vi "Refresh Hierarchy View.vi"(8 "Error in":errorcluster caption="Error in (no error)", 11 "Tree":refnum<vi>) -> (0 "Error out":errorcluster)   [LabVIEW 2018]
uses:
  TypeDef/Refresh Hierarchy View - States.ctl
  TypeDef/BOM Table Raw Items.ctl
  TypeDef/FIlter.ctl
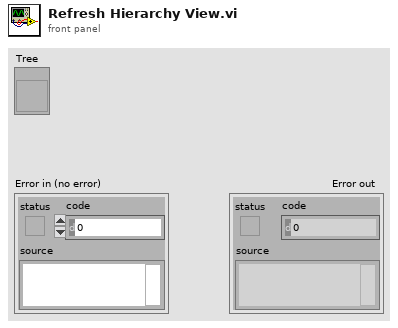
[diagram p1: front panel]
types:
  T1 = typedef "BOM Table Raw Items.ctl" = cluster{"id":i32, "Full PN":string, "External Part Number":string, "Item description":string, "Part Number":string, "Revision":string, "Containing":cluster{"id":i32, "value":string}[], "Contained by":cluster{"id":i32, "value":string}[], "Part of a set":cluster{"id":i32}[]}
  T2 = typedef "Refresh Hierarchy View - States.ctl" = enum16{"Defer Panel Updates", "Cleanup Tree", "Set Up Columns", "Ping API", "GET BOM Rows", "Populate Table", "Adjust Column Width", "Release Panel Updates", "Report Error", "Exit"}
  T3 = typedef "FIlter.ctl" = cluster{"Field Name":string, "Filter Type":string, "Filter Value":string}
  T4 = cluster{"ID":i32, "Item":cluster{"id":i32}[], "Contains":cluster{"id":i32}[], "Amount of Times":string, "Length (mm)":string}
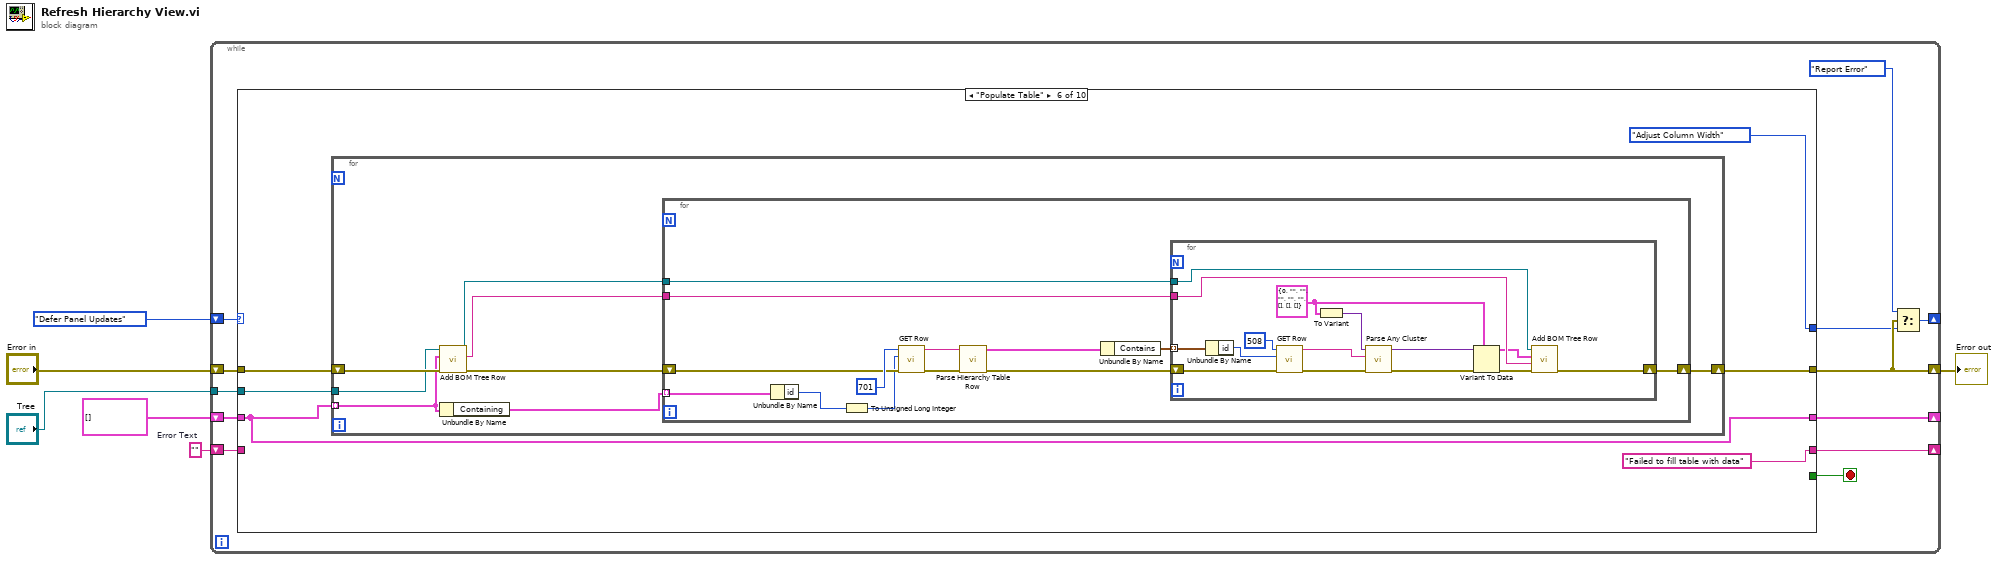
[diagram p0: block diagram]
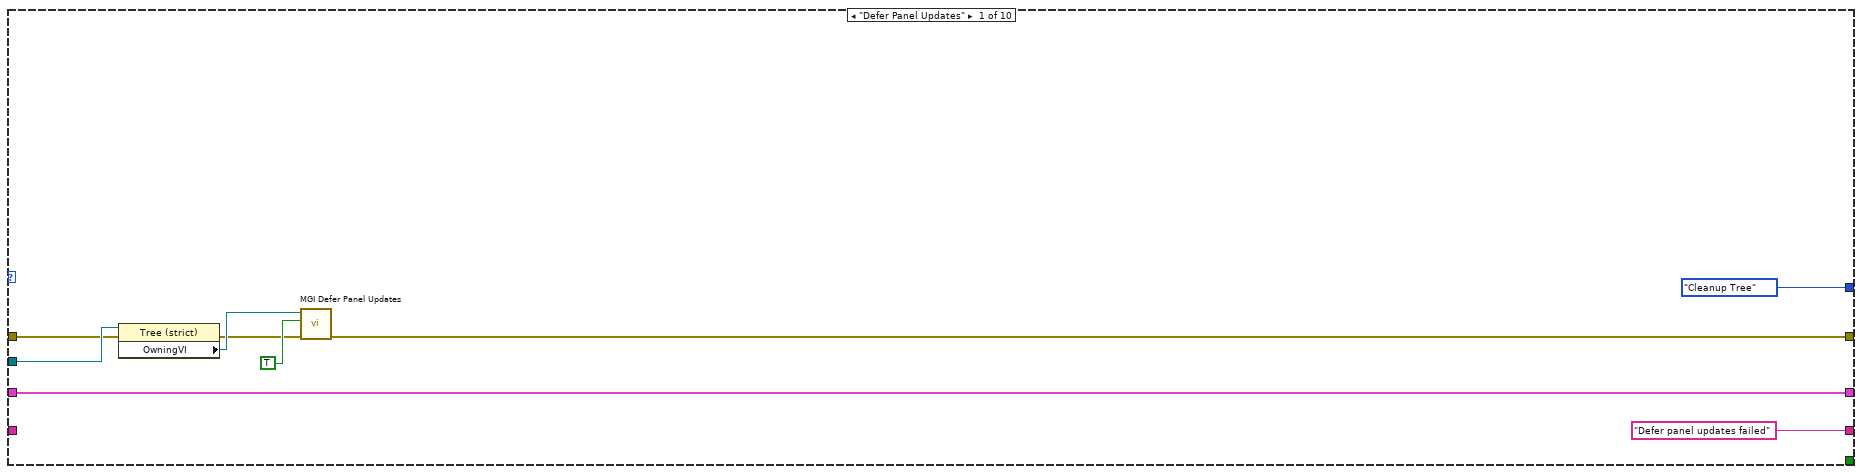
[diagram p2: hidden frame]
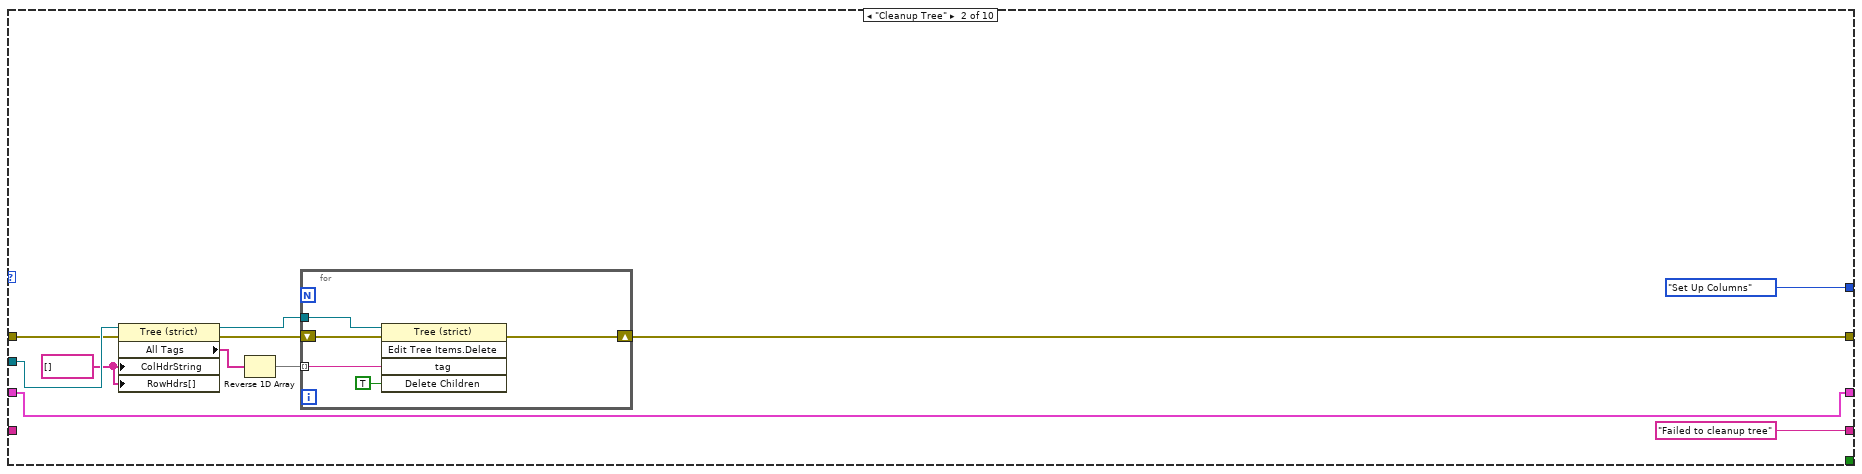
[diagram p3: hidden frame]
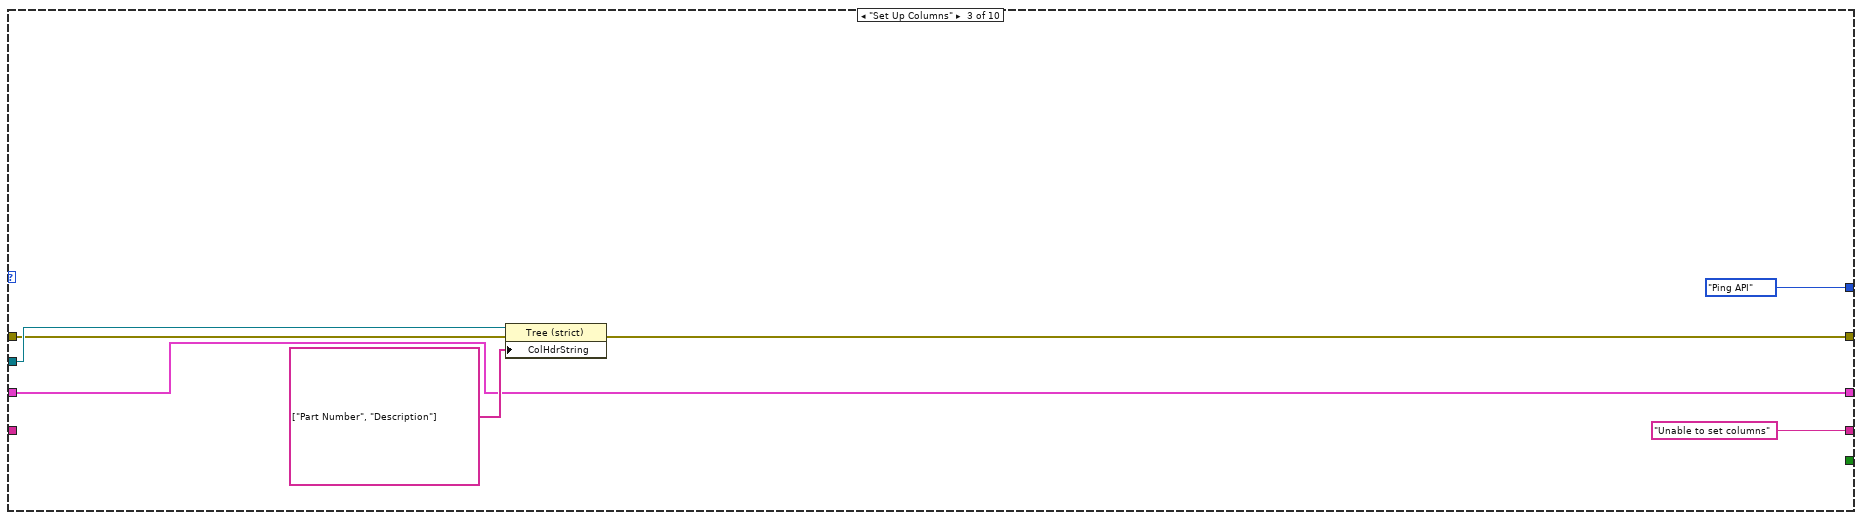
[diagram p4: hidden frame]
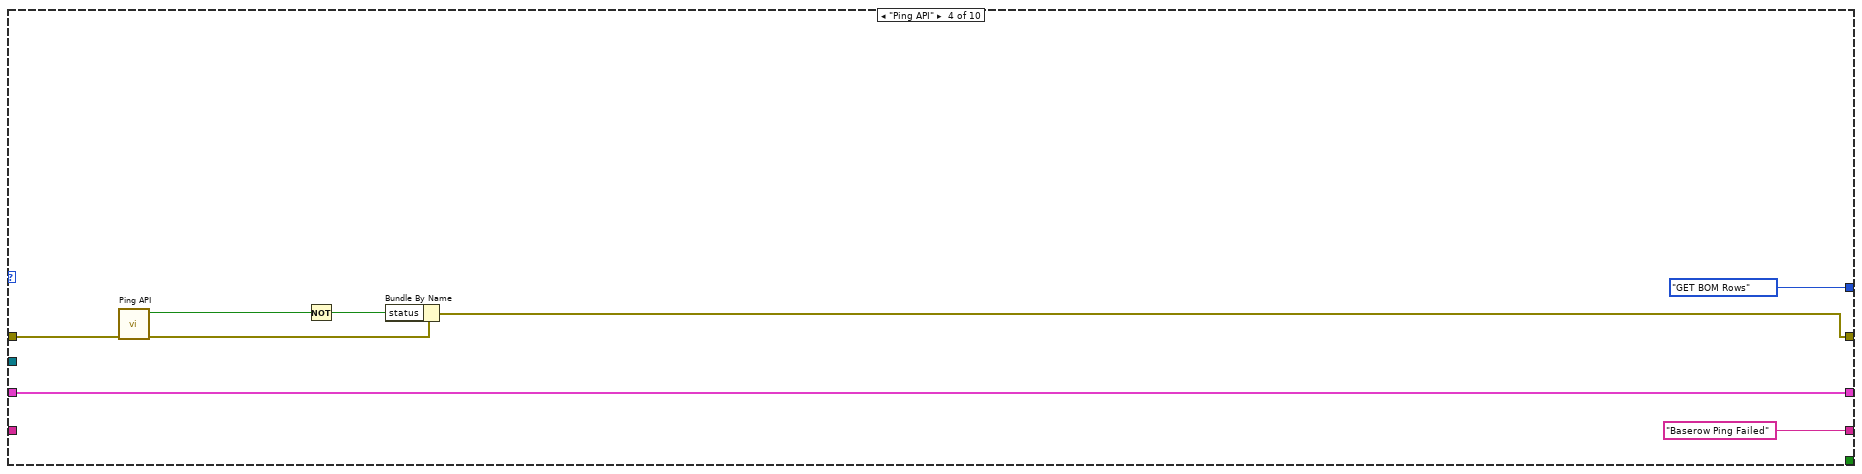
[diagram p5: hidden frame]
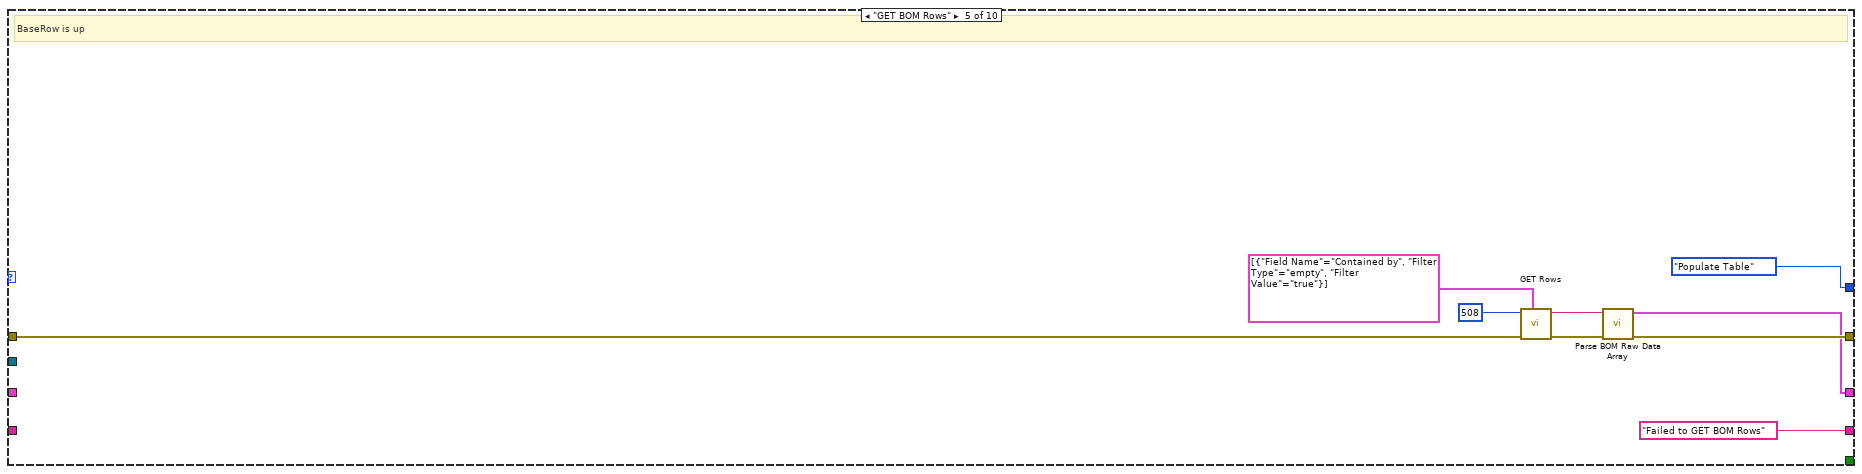
[diagram p6: hidden frame]
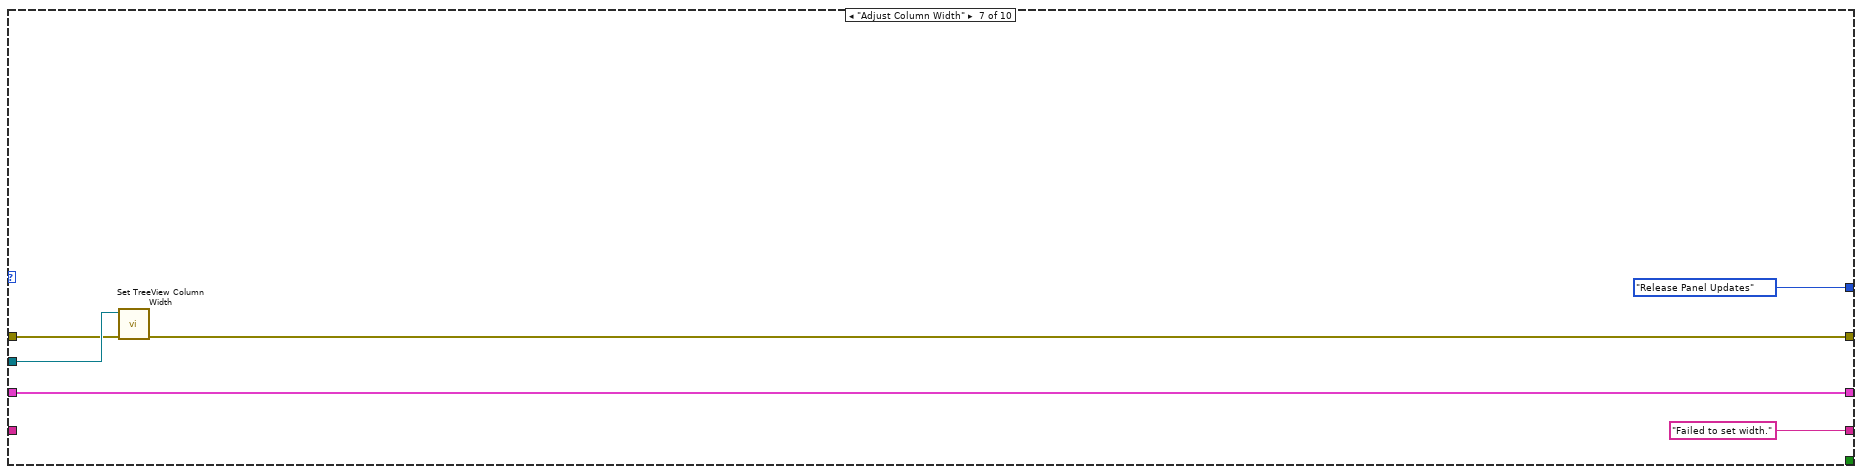
[diagram p7: hidden frame]
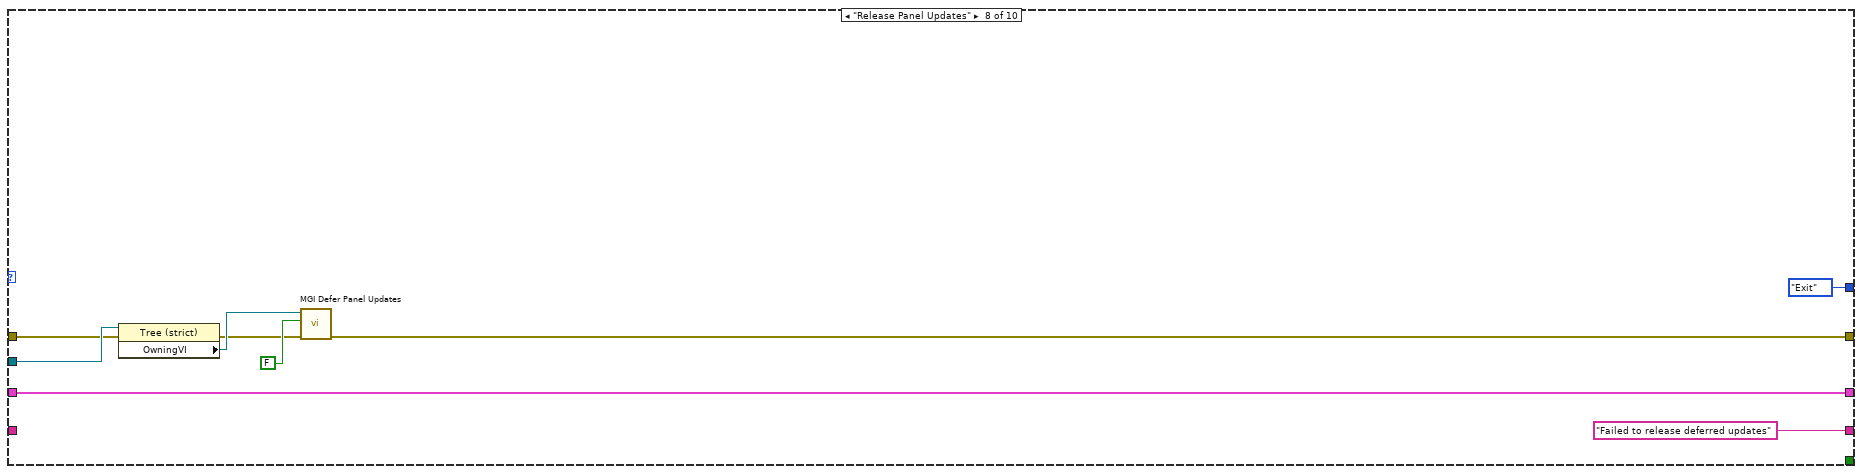
[diagram p8: hidden frame]
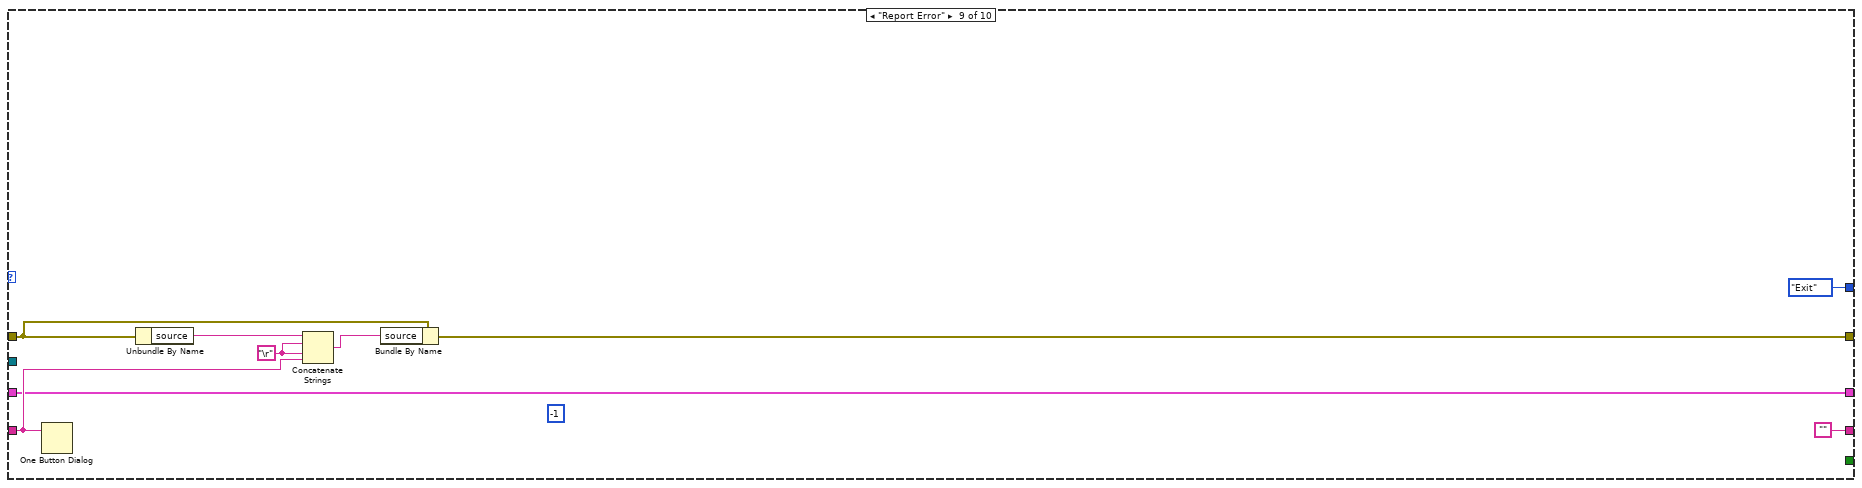
[diagram p9: hidden frame]
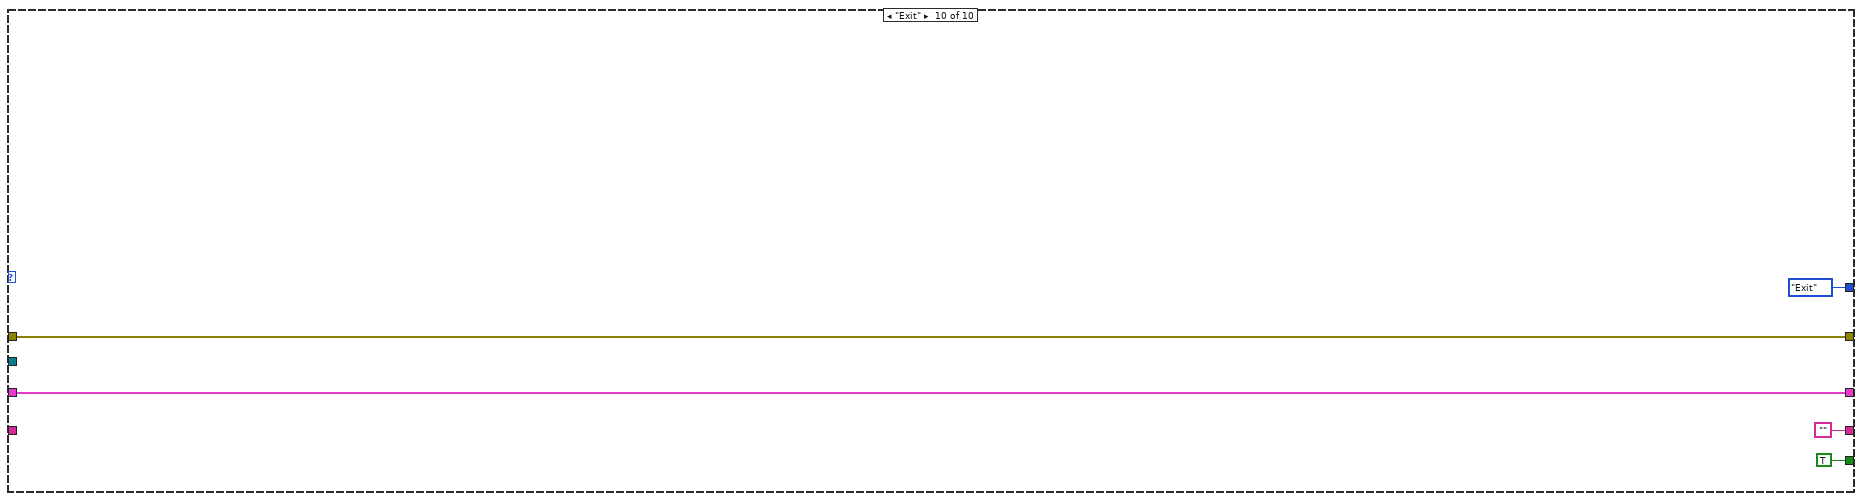
[diagram p10: hidden frame]
diagram:
  w3 = ""  # Error Text
  n1 = while {
    shift-right: [w13] -> w6
    shift-left: "Error in" -> [w17]
    tunnel: "Tree" -> [w14]
    shift-right: [w11] -> _
    shift-left: Refresh_Hierarchy_View_-_States."Defer Panel Updates" -> [w18]
    shift-right: [w9] -> _
    shift-left: w3 -> [w15]
    shift-right: [w8] -> _
    shift-left: T1[] [] ("BOM Items Raw Data") -> [w7]
    stop <- w16 stop-if-true
    n2 = case shown="\"Populate Table\"" w18 {
      tunnel: [w24 w32 w49 w56 w62 w71 w111 w121 w132 w137] -> w13
      tunnel: w17 -> [w22 w37 w48 w58 w65 w70 w110 w119 w131 w137]
      tunnel: [_ _ _ _ _ _ _ _ _ TRUE] -> w16
      tunnel: w15 -> [_ _ _ _ _ _ _ _ w128 _]
      tunnel: w14 -> [w27 w38 w50 _ _ w72 w112 w124 _ _]
      tunnel: [Refresh_Hierarchy_View_-_States."Cleanup Tree" Refresh_Hierarchy_View_-_States."Set Up Columns" Refresh_Hierarchy_View_-_States."Ping API" Refresh_Hierarchy_View_-_States."GET BOM Rows" Refresh_Hierarchy_View_-_States."Populate Table" Refresh_Hierarchy_View_-_States."Adjust Column Width" Refresh_Hierarchy_View_-_States."Release Panel Updates" Refresh_Hierarchy_View_-_States."Exit" Refresh_Hierarchy_View_-_States."Exit" Refresh_Hierarchy_View_-_States."Exit"] -> w12
      tunnel: ["Defer panel updates failed" "Failed to cleanup tree" "Unable to set columns" "Baserow Ping Failed" "Failed to GET BOM Rows" "Failed to fill table with data" "Failed to set width." "Failed to release deferred updates" "" ""] -> w9
      tunnel: [w19 w28 w44 w51 w59 w68 w115 w117 w125 w134] -> w8
      tunnel: w7 -> [w19 w28 w44 w51 _ w68 w115 w117 w125 w134]
      frame "Defer Panel Updates" {
        n3 = property class="Tree (strict)"(reference=w27, error in=w22) -> (error out=w23:errorcluster, "OwningVI"=w26:refnum<vi>)  [unwired: 1 out]
        n4 = call <userlib>:"MGI Defer Panel Updates.vi"("Error In"=w23, "Defer Updates?"=TRUE, "VI Reference (Caller)"=w26) -> ("Error Out"=w24:errorcluster)  [unwired: 8 in]
      }
      frame "Cleanup Tree" {
        w31 = string[] [] ("Column Header Strings[]")
        n5 = property class="Tree (strict)"(reference=w38, error in=w37, "ColHdrString"=w31, "RowHdrs[]"=w31) -> (reference out=w35:refnum<vi>, error out=w33:errorcluster, "All Tags"=w36:string[])
        n6 = Reverse 1D Array(array=w36) -> (reversed array=w34:string[])
        n7 = for {
          tunnel: w35 -> [w43]
          tunnel: w34 -> [w42] mode=indexing
          shift-right: [w39] -> w32
          shift-left: w33 -> [w40]
          n8 = invoke class="Tree (strict)" method="Edit Tree Items.Delete"(reference=w43, error in=w40, "tag"=w42, "Delete Children"=TRUE ("Delete Children?")) -> (error out=w39:errorcluster)  [unwired: 1 in, 4 out]
        }
      }
      frame "Set Up Columns" {
        n9 = property class="Tree (strict)"(reference=w50, error in=w48, "ColHdrString"=string[] ["Part Number", "Description"] ("Column Header Strings[]")) -> (error out=w49:errorcluster)  [unwired: 1 out]
      }
      frame "Ping API" {
        n10 = call "Ping API.vi"("Error in"=w58) -> ("Error out"=w57:errorcluster, "Connection OK"=w55:bool)  [unwired: 9 in]
        n11 = Not(x=w55) -> (.not. x?=w52:bool)
        n12 = Bundle By Name(cluster=w57, "status"=w52) -> (w56:errorcluster)
      }
      frame "GET BOM Rows" {
        # "BaseRow is up"
        n13 = call "GET Rows.vi"("Filters"=T3[] [{"Field Name"="Contained by", "Filter Type"="empty", "Filter Value"="true"}], "Error in"=w65, "Table ID"=u32 508) -> ("Error out"=w63:errorcluster, "Rows Array JSON"=w64:string)  [unwired: 7 in]
        n14 = call "Parse BOM Raw Data Array.vi"("Error in"=w63, "BOM JSON String"=w64) -> ("Error out"=w62:errorcluster, "BOM Items Raw Data"=w59:T1[])  [unwired: 8 in]
      }
      frame "Populate Table" {
        n15 = for {
          tunnel: w72 -> [w80]
          shift-right: [w78] -> w71
          shift-left: w70 -> [w81]
          tunnel: w68 -> [w75] mode=indexing
          n16 = call "Add BOM Tree Row.vi"("error in (no error)"=w81, "BOM Table Raw Items"=w75, "TreeControl in"=w80) -> ("error out"=w79:errorcluster, "New Item Tag"=w76:string, "TreeControl out"=w77:refnum<vi>)  [unwired: 6 in]
          n17 = Unbundle By Name(w75) -> ("Containing"=w74:cluster{"id":i32, "value":string}[])
          n18 = for {
            shift-right: [w84] -> w78
            shift-left: w79 -> [w87]
            tunnel: w74 -> [w93] mode=indexing
            tunnel: w77 -> [w86]
            tunnel: w76 -> [w85]
            n19 = Unbundle By Name(w93) -> ("id"=w83:i32)
            n20 = To Unsigned Long Integer(number=w83) -> (unsigned 32bit integer=w82:u32)
            n21 = call "GET Row.vi"("Error in"=w87, "Row ID"=w82, "Table ID"=u32 701) -> ("Error out"=w91:errorcluster, "Rows Array JSON"=w92:string)  [unwired: 7 in]
            n22 = call "Parse Hierarchy Table Row.vi"("Error in"=w91, "Rows Array JSON"=w92) -> ("Error out"=w88:errorcluster, "data"=w90:T4)  [unwired: 8 in]
            n23 = Unbundle By Name(w90) -> ("Contains"=w89:cluster{"id":i32}[])
            n24 = for {
              tunnel: w89 -> [w109] mode=indexing
              shift-right: [w96] -> w84
              shift-left: w88 -> [w106]
              tunnel: w86 -> [w105]
              tunnel: w85 -> [w104]
              w103 = T1 {"id"=0, "Full PN"="", "External Part Number"="", "Item description"="", "Part Number"="", "Revision"="", "Containing"=[], "Contained by"=[], "Part of a set"=[]}
              n25 = Unbundle By Name(w109) -> ("id"=w108:i32)
              n26 = call "GET Row.vi"("Error in"=w106, "Row ID"=w108, "Table ID"=u32 508) -> ("Error out"=w99:errorcluster, "Rows Array JSON"=w102:string)  [unwired: 7 in]
              n27 = To Variant(anything=w103) -> (Variant=w101:variant)
              n28 = call "Parse Any Cluster.vi"("error in (no error)"=w99, "JSON In"=w102, "Cluster in"=w101) -> ("error out"=w95:errorcluster, "Cluster out"=w100:variant)  [unwired: 7 in]
              n29 = Variant To Data(error in=w95, type=w103, Variant=w100) -> (data=w98:T1, error out=w97:errorcluster)
              n30 = call "Add BOM Tree Row.vi"("error in (no error)"=w97, "Parent Tag"=w104, "BOM Table Raw Items"=w98, "TreeControl in"=w105) -> ("error out"=w96:errorcluster)  [unwired: 5 in, 2 out]
            }
          }
        }
      }
      frame "Adjust Column Width" {
        n31 = call "Set TreeView Column Width.vi"("error in (no error)"=w110, "TreeControl in"=w112) -> ("error out"=w111:errorcluster)  [unwired: 9 in]
      }
      frame "Release Panel Updates" {
        n32 = property class="Tree (strict)"(reference=w124, error in=w119) -> (error out=w120:errorcluster, "OwningVI"=w123:refnum<vi>)  [unwired: 1 out]
        n33 = call <userlib>:"MGI Defer Panel Updates.vi"("Error In"=w120, "Defer Updates?"=FALSE, "VI Reference (Caller)"=w123) -> ("Error Out"=w121:errorcluster)  [unwired: 8 in]
      }
      frame "Report Error" {
        w129 = "\r"
        (unwired) -1 ("code")
        n34 = One Button Dialog(message=w128) -> ()  [unwired: 1 in, 1 out]
        n35 = Unbundle By Name(w131) -> ("source"=w130:string)
        n36 = Concatenate Strings(w130, w129, w129, w128) -> (w127:string)
        n37 = Bundle By Name(cluster=w131, "source"=w127) -> (w132:errorcluster)
      }
      frame "Exit" {
      }
    }
    n38 = Select(t=Refresh_Hierarchy_View_-_States."Report Error", s=w13, f=w12) -> (s? t:f=w11:T2)
  }
  "Error out" <- w6
